vi "Calculate Output Power.vi"(8 "error in (no error)":errorcluster, 9 "load impedance":dbl, 11 "waveforms":waveform(dbl)[](array[waveform])) -> (0 "error out":errorcluster, 3 "output power":dbl[](array[numeric]))   [LabVIEW 2023]
uses:
  <vilib>/addons/Sound and Vibration/svt_Level/SVL RMS Level (N Ch).vi
  <vilib>/addons/Sound and Vibration/svt_Level/SoundVib_VibrationLevel.lvlib
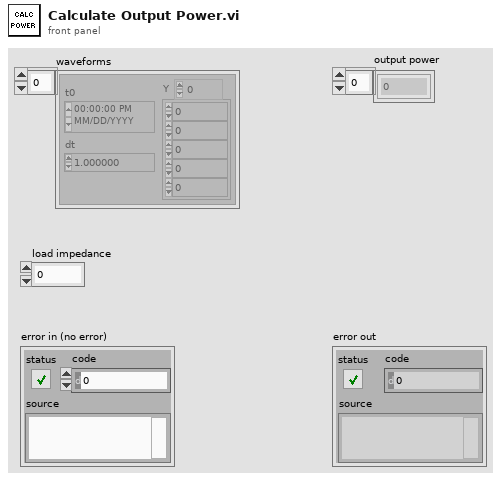
[diagram p1: front panel]
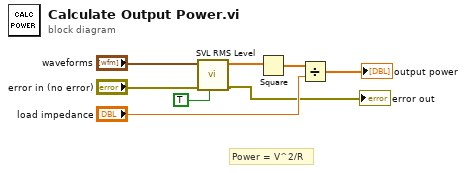
[diagram p0: block diagram]
diagram:
  # "Power = V^2/R"
  n1 = call-poly <vilib>:"SVL RMS Level.vi"("restart averaging (F)"=TRUE, "error in (no error)"="error in (no error)", "scaled signals [EU]"="waveforms") -> ("error out"=→"error out":errorcluster, "RMS levels [EU rms]"=w7:dbl[])  [unwired: 6 in, 1 out]
  n2 = Square(x=w7) -> (x^2=w6:dbl[])
  n3 = Divide(x=w6, y="load impedance") -> (x/y=→"output power":dbl[])
